vi "SaveMesLog.vi"(9 "String":string, 10 "SN":string) -> ()   [LabVIEW 2017]
panel:
  in  "错误输入":errorcluster
  out "错误输出 2":errorcluster caption="错误输出"
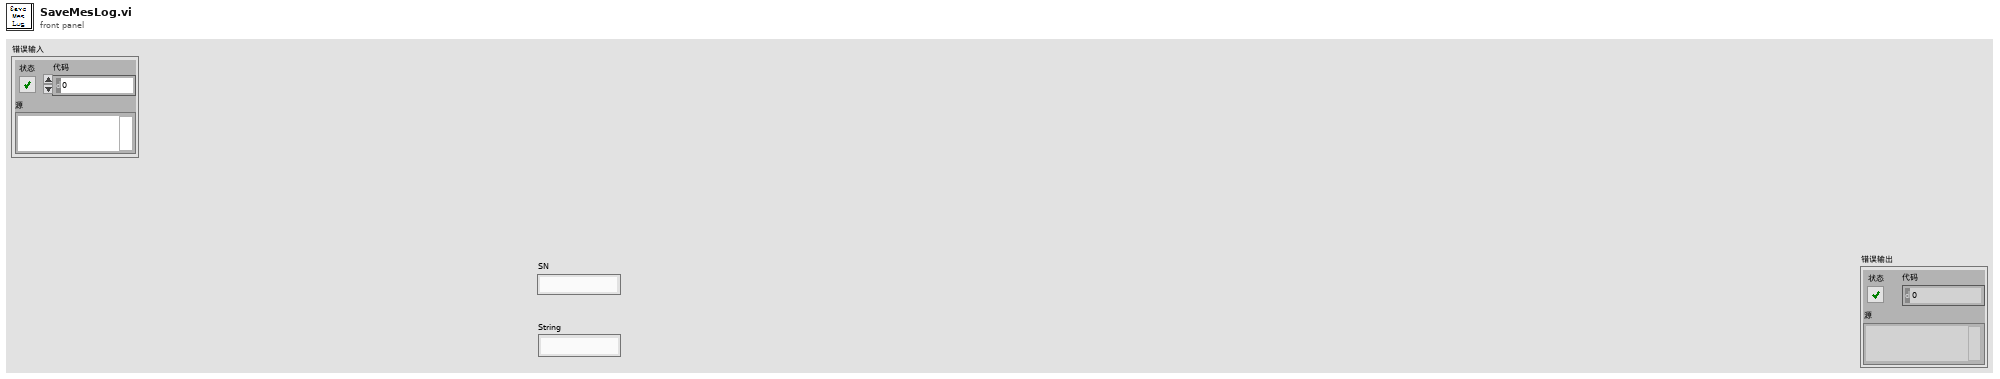
[diagram p1: front panel]
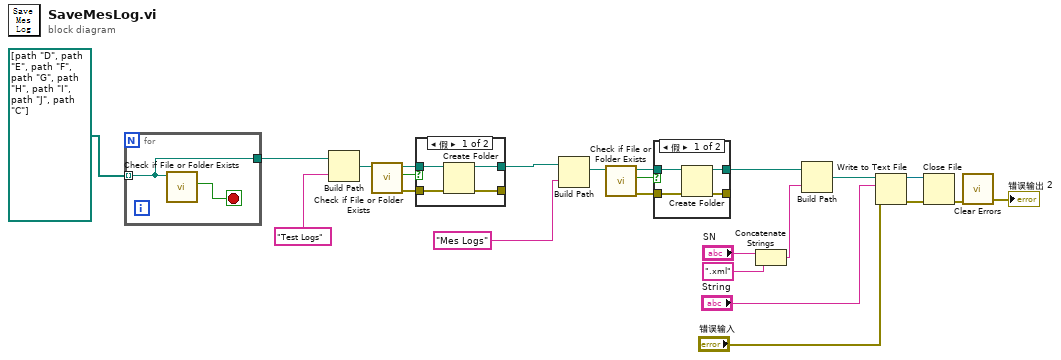
[diagram p0: block diagram]
diagram:
  n1 = for {
    tunnel: path[] [path "D:/", path "E:/", path "F:/", path "G:/", path "H:/", path "I:/", path "J:/", path "C:/"] -> [w25] mode=indexing
    tunnel: [w25] -> w19
    stop <- w26 stop-if-true
    n2 = call <vilib>:"Check if File or Folder Exists.vi"("path"=w25) -> ("file or folder exists?"=w26:bool)  [unwired: 8 in, 2 out]
  }
  n3 = Build Path(base path=w19, name or relative path="Test Logs") -> (appended path=w17:path)
  n4 = call <vilib>:"Check if File or Folder Exists.vi"("path"=w17) -> ("error out"=w23:errorcluster, "file or folder exists?"=w24:bool, "dup path"=w22:path)  [unwired: 8 in]
  n5 = case shown="假" w24 {
    tunnel: w23 -> [w29 w31]
    tunnel: w22 -> [w30 w32]
    tunnel: [w27 w32] -> w21
    tunnel: [w28 w31] -> _
    frame False {
      n6 = Create Folder(path (use dialog)=w30, error in=w29) -> (created path=w27:path, error out=w28:errorcluster)  [unwired: 1 in, 1 out]
    }
    frame True {
    }
  }
  n7 = Build Path(base path=w21, name or relative path="Mes Logs") -> (appended path=w13:path)
  n8 = call <vilib>:"Check if File or Folder Exists.vi"("path"=w13) -> ("error out"=w15:errorcluster, "file or folder exists?"=w14:bool, "dup path"=w16:path)  [unwired: 8 in]
  n9 = case shown="假" w14 {
    tunnel: w15 -> [w35 w37]
    tunnel: w16 -> [w36 w38]
    tunnel: [w33 w38] -> w11
    tunnel: [w34 w37] -> _
    frame False {
      n10 = Create Folder(path (use dialog)=w36, error in=w35) -> (created path=w33:path, error out=w34:errorcluster)  [unwired: 1 in, 1 out]
    }
    frame True {
    }
  }
  n11 = Concatenate Strings("SN", ".xml" ("字符串")) -> (w4:string)
  n12 = Build Path(base path=w11, name or relative path=w4) -> (appended path=w3:path)
  n13 = Write to Text File(file (use dialog)=w3, text="String", error in="错误输入") -> (refnum out=w6:refnum<file>, error out=w5:errorcluster)  [unwired: 1 in, 1 out]
  n14 = Close File(refnum=w6, error in=w5) -> (error out=w9:errorcluster)  [unwired: 1 out]
  n15 = call <vilib>:"Clear Errors.vi"("error in (no error)"=w9) -> ("error out"=→"错误输出 2":errorcluster)  [unwired: 5 in, 1 out]
